vi "HEWH Save Final Data.vi"(0 "RTD Max Min Array":dbl[][](array[numeric]), 5 "No Path?":bool, 9 "Final Data Cluster":T2={"Scan Rate Adjust"=1000.0, "Draw Count"=0, "Test Patten Setup"={"Dispense Times"=[0.0, 3600.0, 7200.0, 10800.0, 14400.0, 18000.0], "Total Gallons Schedule"=[10.72, 10.72, 10.72, 10.72, 10.72, 10.72], "Flow Rate Schedule "=[3.0, 3.0, 3.0, 3.0, 3.0, 3.0], "Incoming Water Temperature"=[58.0, 58.0, 58.0, 58.0, 58.0, 58.0], "PreDraw Pattern"=[], "24 Hour PreDraw"=enum."Zero Pre-Draws", "Pre-Draw Until?"=[], "Purge Until Cutout"=FALSE, "Heating Flag"=FALSE, "PRAT/RLT Sequence"=[]}, "Condition Cluster Output"={"Condition #1"=FALSE, "Condition #2"=FALSE, "Special Last Draw (HU Test)"=FALSE, "RTD Out Temperature <="=0.0, "Condition #3"=FALSE, "Mean Tank Temperature <="=0.0, "Condition #4"=FALSE, "Decrease Outlet Temperature \nBy (RTD Out)"=0.0, "Condition #5"=FALSE, "Condition #6"=FALSE, "Time (Seconds)"=0.0, "Condition #7"=FALSE, "Condition #8"=FALSE, "Draw Until Condition"={"UE"=FALSE, "LE"=FALSE, "COMP"=FALSE, "FANS"=FALSE}, "Condition #9"=FALSE}, "HEWH Specific DAQ"={"HEWH Data"={"HEWH Standard"={"Voltage (Volts)"=-1.0, "Current (Amps)"=-1.0, "Power (Watts)"=-1.0, "WattHours (Wh)"=-1.0, "TC Tree (AVG)"=0.0, "Flow Rate (GPM)"=0.0, "Gallons (Gal)"=0.0, "RTD Out (Deg F)"=0.0, "RTD In (Deg F)"=0.0, "RTD Amb (Deg F)"=0.0, "TC Down"=0.0, "UE Event Lead"=0, "LE Event Lead"=0, "TC Tree Array"=[]}, "PRAT"={"Power (Watts) A"=0.0, "Power (Watts) B"=0.0, "Power (Watts) C"=0.0, "Power (Watts) D"=0.0, "TC1"=0.0, "TC2"=0.0, "TC3"=0.0, "TC4"=0.0, "WattHours (Wh) A"=0.0, "WattHours (Wh) B"=0.0, "WattHours (Wh) C"=0.0, "WattHours (Wh) D"=0.0, "Ambient"=0.0, "Extra Temp"=0.0}, "Additional Power Data"={"Vthd"=0.0, "Frequency (Hz)"=0.0, "Apparent Power (VA)"=0.0, "Power Factor"=0.0, "Current Crest Factor"=0.0, "Voltage Crest Factor"=0.0, "Integration Time (sec)"=0.0}}, "Intellif Valve % Open"=0.0, "Power State"={"UE"=FALSE, "LE"=FALSE, "COMP"=FALSE, "FANS"=FALSE}, "Power Analyzer"=enum."APLUS", "Intellifaucet Configuration"=enum."DRK375,STATION3,1/2\"HOSE"}, "Test Output Data"={"PreDraw Data Table"=[], "Data Table"=[], "MW100 TC Headers"=[]}, "Calc and Calibration"={"Mean SD Var Max Min Array"=[], "Draw Statistics (DBL)"=[], "Calibration Coefficients DBL"=[], "Start Gallons"=0.0, "Starting Temp Decline"=0.0, "K-Factor (Intellifaucet)"=0.0, "All Draw Stats"=[], "RTD Terminate Value"=0.0}, "Current Draw Time"=0.0, "LV Program"=enum."HEWH", "Station ID"=enum."A"} {"Test Patten Setup"."PRAT/RLT Sequence"."Time" format="%<%H:%M:%S>t"; "Test Patten Setup"."Incoming Water Temperature" format="%.2f"; "Test Patten Setup"."Flow Rate Schedule" format="%.2f"; "Test Patten Setup"."Total Gallons Schedule" format="%.2f"; "Test Patten Setup"."Dispense Times" format="%<%H:%M:%S>t"}, 11 "error in (no error)":errorcluster, 12 "Save File Path":path, 14 "Sofware Version":T1) -> (4 "Data With Header":string[][](array[string]), 15 "error out":errorcluster)   [LabVIEW 2016]
uses:
  Type Definitions/HEWH Power Data.ctl
  Type Definitions/HEWH PreDraw.ctl
  Type Definitions/HEWH Draw Pattern Setup.ctl
  Type Definitions/HEWH Power Elements.ctl
  Type Definitions/HEWH Termination Condition Cluster.ctl
  Type Definitions/HEWH Output Information.ctl
  Utility/Custom Pallet Controls/Custom Pallet String.ctl
  Utility/Type Definitions/UTILITY Power Analyzer.ctl
  Custom Instrument Control/Intellifaucet/Type Definitions/INTELLIFAUCET Tested Flowrate Scenarios.ctl
  Utility/Save File/File Setup (Public)/Type Definition/Save File HEWH Heating Control Mode.ctl
  Utility/Save File/File Setup.lvlib
  Type Definitions/PRAT Test.ctl
  Type Definitions/HEWH Calc and Calibration.ctl
  Utility/Save File/File Setup (Public)/Type Definition/Save File DOE LabView Program.ctl
  Custom Instrument Control/MW100/Type Definitions/Station ID Selector.ctl
  Draw Water Specific/Type Definitions/Terminate Draw Conditions.ctl
  Type Definitions/HEWH Start Conditions.ctl
  Draw Water Specific/Type Definitions/Check Special Condtions.ctl
  Type Definitions/HEWH Draw Flag ENUM.ctl
  Draw Water Specific/Type Definitions/HEWH Special Condition Check.ctl
panel:
  # "Select Only One Condition"
  # "Just Draw Water!"
  # "Condition #1"
  # "Draw Until Any Heat Source"
  # "Condition #2"
  # "Start Dispense Pattern"
  # "Draw Until Specific Heat Source"
  # "Condition #3"
  # "Dispense PRAT Sequence"
  # "Not Working"
  # "Condition #4"
  # "Condition #5"
  # "Condition #6"
  # "Draw Pattern Setup (24 Hour)"
  # "Pre-Draw Items"
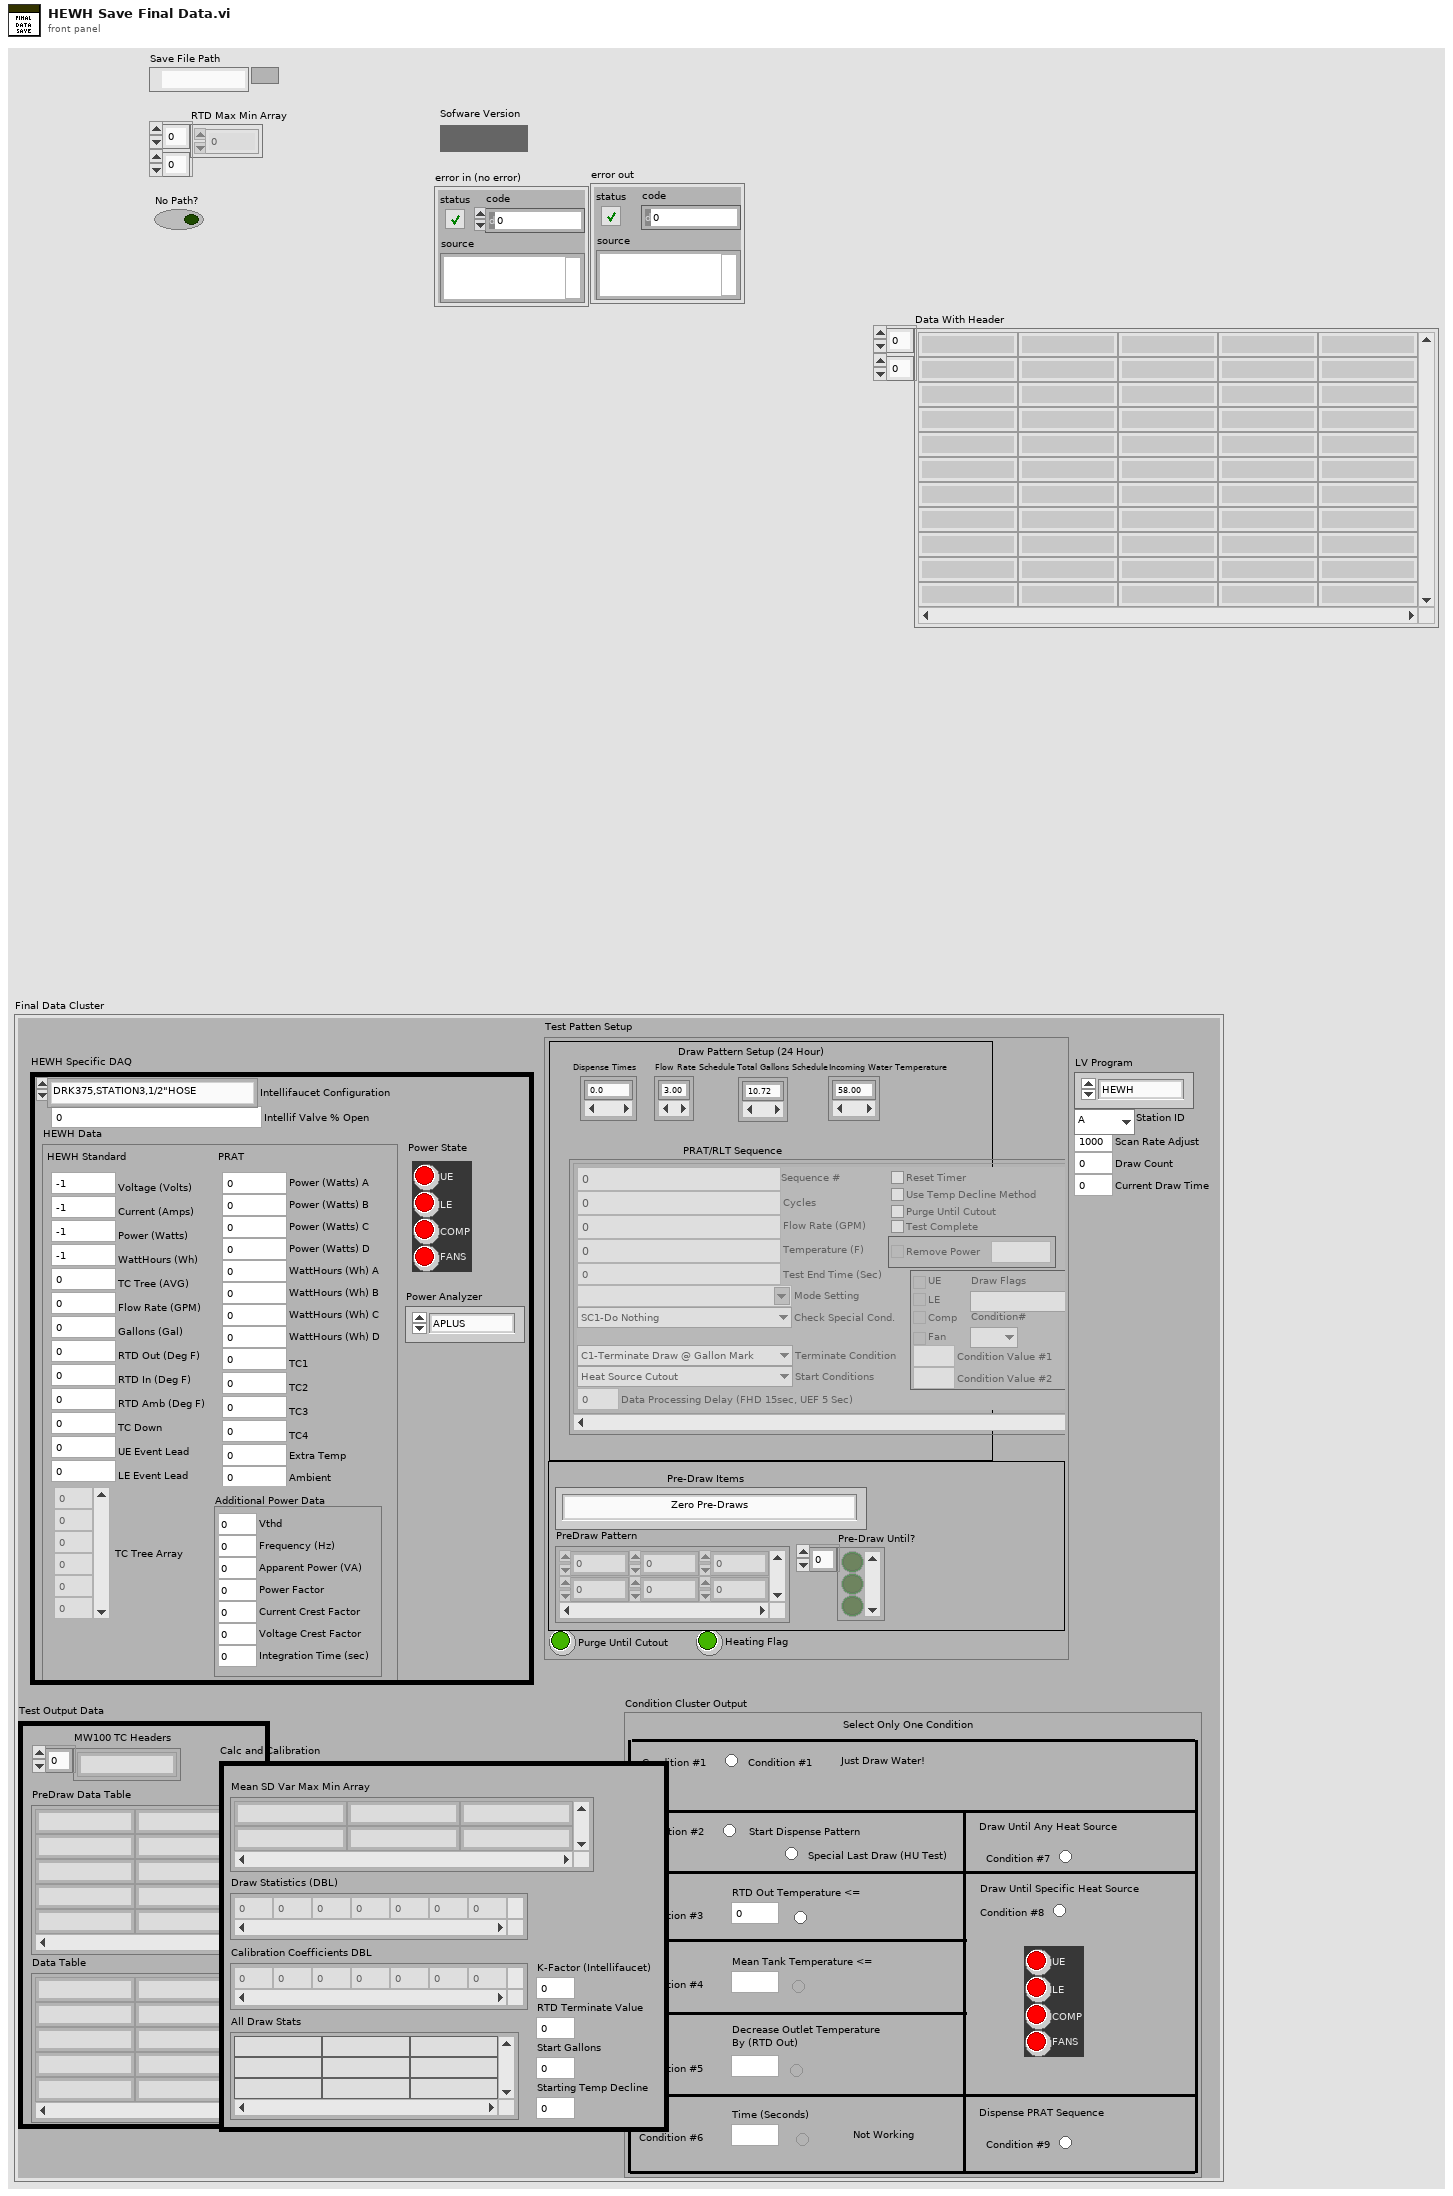
[diagram p1: front panel]
types:
  T1 = typedef "Custom Pallet String.ctl" = string
  T2 = typedef "HEWH Output Information.ctl" = cluster{"Scan Rate Adjust":dbl, "Draw Count":i32, "Test Patten Setup":T3, "Condition Cluster Output":T12, "HEWH Specific DAQ":cluster{"HEWH Data":T14, "Intellif Valve % Open":dbl, "Power State":T13, "Power Analyzer":T15, "Intellifaucet Configuration":T16}, "Test Output Data":cluster{"PreDraw Data Table":string[][], "Data Table":string[][], "MW100 TC Headers":string[]}, "Calc and Calibration":T17, "Current Draw Time":dbl, "LV Program":T18, "Station ID":T19}
  T3 = typedef "HEWH Draw Pattern Setup.ctl" = cluster{"Dispense Times":dbl[], "Total Gallons Schedule":dbl[], "Flow Rate Schedule ":dbl[], "Incoming Water Temperature":dbl[], "PreDraw Pattern":dbl[][], "24 Hour PreDraw":T4, "Pre-Draw Until?":bool[], "Purge Until Cutout":bool, "Heating Flag":bool, "PRAT/RLT Sequence":T5[]}
  T4 = typedef "HEWH PreDraw.ctl" = enum16{"Zero Pre-Draws", "One Pre- Draws", "Two Pre-Draws", "Three Pre-Draws", ""}
  T5 = typedef "PRAT Test.ctl" = cluster{"Sequence #":dbl, "Cycles":i32, "Mode Setting":T6, "Flow Rate (GPM)":dbl, "Temperature (F)":dbl, "Reset Timer":bool, "Use Temp Decline Method":bool, "Terminate Condition":T7, "Condition Value #1":dbl, "UE":bool, "LE":bool, "Comp":bool, "Fan":bool, "Test End Time (Sec)":dbl, "Purge Until Cutout":bool, "Start Conditions":T8, "Condition Value #2":dbl, "Remove Power":bool, "Time":dbl, "Check Special Cond.":T9, "Condition#":T10, "Draw Flags":T11, "Data Processing Delay (FHD 15sec, UEF 5 Sec)":dbl, "Test Complete":bool}
  T6 = typedef "File Setup.lvlib/Save File HEWH Heating Control Mode.ctl" = string
  T7 = typedef "Terminate Draw Conditions.ctl" = enum16{"C1-Terminate Draw @ Gallon Mark", "C2-Special Last Draw (HU Test)", "C3-RTD Out <=", "C4-Mean Tank Temp <=", "C5-Decrease RTD Out (Deg F)", "C6-Time (Seconds)", "C7-Until Any Heat Source", "C8-Specific Heat Source", "C9-Do Nothing"}
  T8 = typedef "HEWH Start Conditions.ctl" = enum16{"Heat Source Cutout", "At Time (Seconds)", "Every X (Seconds)", "T2 >= X° Below Setpoint", "Seconds From Complete", "Wait for LE & Comp Cutout", "Wait for Comp Cutout", "Wait for LE Cutout", "Wait for UE Cutout"}
  T9 = typedef "Check Special Condtions.ctl" = enum16{"SC1-Do Nothing", "SC2-Check Heat Source (On-C2/Off-C1)", "SC3-Check Skip Condition", "SC4-Check Heat Source ON/Fail"}
  T10 = typedef "HEWH Special Condition Check.ctl" = enum16{"N/A", "C1", "C2", "Reset/Fail", "Skip Draw Sequence"}
  T11 = typedef "HEWH Draw Flag ENUM.ctl" = enum16{"N/A", "None(0)", "Sml(1)", "Med(2)", "SmlMed(3)", "Lrg(4)", "SmlLrg(5)", "MedLrg(6)", "SmlMedLrg(7)"}
  T12 = typedef "HEWH Termination Condition Cluster.ctl" = cluster{"Condition #1":bool, "Condition #2":bool, "Special Last Draw (HU Test)":bool, "RTD Out Temperature <=":dbl, "Condition #3":bool, "Mean Tank Temperature <=":dbl, "Condition #4":bool, "Decrease Outlet Temperature \nBy (RTD Out)":dbl, "Condition #5":bool, "Condition #6":bool, "Time (Seconds)":dbl, "Condition #7":bool, "Condition #8":bool, "Draw Until Condition":T13, "Condition #9":bool}
  T13 = typedef "HEWH Power Elements.ctl" = cluster{"UE":bool, "LE":bool, "COMP":bool, "FANS":bool}
  T14 = typedef "HEWH Power Data.ctl" = cluster{"HEWH Standard":cluster{"Voltage (Volts)":dbl, "Current (Amps)":dbl, "Power (Watts)":dbl, "WattHours (Wh)":dbl, "TC Tree (AVG)":dbl, "Flow Rate (GPM)":dbl, "Gallons (Gal)":dbl, "RTD Out (Deg F)":dbl, "RTD In (Deg F)":dbl, "RTD Amb (Deg F)":dbl, "TC Down":dbl, "UE Event Lead":i32, "LE Event Lead":i32, "TC Tree Array":dbl[]}, "PRAT":cluster{"Power (Watts) A":dbl, "Power (Watts) B":dbl, "Power (Watts) C":dbl, "Power (Watts) D":dbl, "TC1":dbl, "TC2":dbl, "TC3":dbl, "TC4":dbl, "WattHours (Wh) A":dbl, "WattHours (Wh) B":dbl, "WattHours (Wh) C":dbl, "WattHours (Wh) D":dbl, "Ambient":dbl, "Extra Temp":dbl}, "Additional Power Data":cluster{"Vthd":dbl, "Frequency (Hz)":dbl, "Apparent Power (VA)":dbl, "Power Factor":dbl, "Current Crest Factor":dbl, "Voltage Crest Factor":dbl, "Integration Time (sec)":dbl}}
  T15 = typedef "UTILITY Power Analyzer.ctl" = enum16{"", "APLUS", "WT210", "WT500", "WT300", "OSI", "Debug", "WT230", "WT300_1", "WT300_2"}
  T16 = typedef "INTELLIFAUCET Tested Flowrate Scenarios.ctl" = enum16{"DRK500,Station1", "DRK375,Lab", "SRK500,Station1,5GPM FR", "DRK375,STATION3,1/2\"HOSE", "DRK500,Station1,downspout", "DRK375,Station3,thruEcocute", "DRK375,Station3,purge", "Build2,2B,Purge", "Global, Purge", "Global, Tank", "DRK250"}
  T17 = typedef "HEWH Calc and Calibration.ctl" = cluster{"Mean SD Var Max Min Array":string[][], "Draw Statistics (DBL)":dbl[][], "Calibration Coefficients DBL":dbl[][], "Start Gallons":dbl, "Starting Temp Decline":dbl, "K-Factor (Intellifaucet)":dbl, "All Draw Stats":string[][], "RTD Terminate Value":dbl}
  T18 = typedef "File Setup.lvlib/Save File DOE LabView Program.ctl" = enum16{"No Name Found", "DOE Stand", "Dishwasher Kitchen", "Portable Stand", "HEWH", "Dryer", "Dryer WILT", "HCC", "PRAT", "HEWH RLT"}
  T19 = typedef "Station ID Selector.ctl" = enum16{"", "A", "B", "C", "D", "Global"}
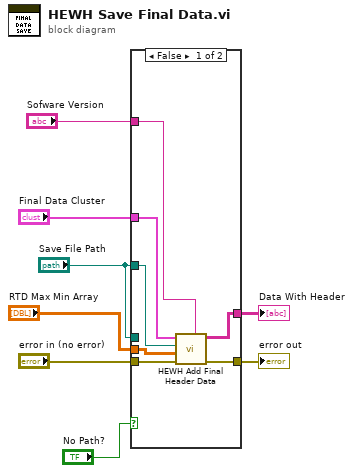
[diagram p0: block diagram]
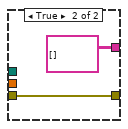
[diagram p2: hidden frame]
diagram:
  n1 = case shown="False" "No Path?" {
    tunnel: "error in (no error)" -> [w9 w17]
    tunnel: [w15 w17] -> w2
    tunnel: "RTD Max Min Array" -> [w14 _]
    tunnel: "Save File Path" -> [w10 _]
    tunnel: "Sofware Version" -> [w13 _]
    tunnel: "Save File Path" -> [_ _]
    tunnel: "Final Data Cluster" -> [w12 _]
    tunnel: [w11 string[][] [] ("Data With Header")] -> w1
    frame False {
      n2 = call "HEWH Add Final Header Data.vi"("Software Version"=w13, "error in (no error)"=w9, "Draw Statistics"=w14, "Save File Path"=w10, "Final Data Cluster"=w12) -> ("error out"=w15:errorcluster, "Data With Header"=w11:string[][])  [unwired: 5 in]
    }
    frame True {
    }
  }
  "error out" <- w2
  "Data With Header" <- w1
